vi "set_size.vi"(8 "error in (no error)":errorcluster, 10 "new size":refnum<class "SpaceVector.lvclass">, 11 "Box in":refnum<class "Box.lvclass">) -> (0 "error out":errorcluster, 3 "Box out":refnum<class "Box.lvclass">)   [LabVIEW 2010, in "Box.lvclass"]
uses:
  Box.lvclass
  SpaceVector/SpaceVector/SpaceVector.lvclass
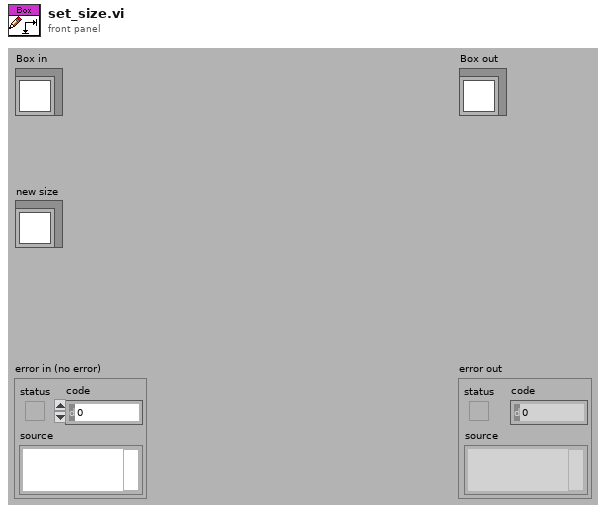
[diagram p1: front panel]
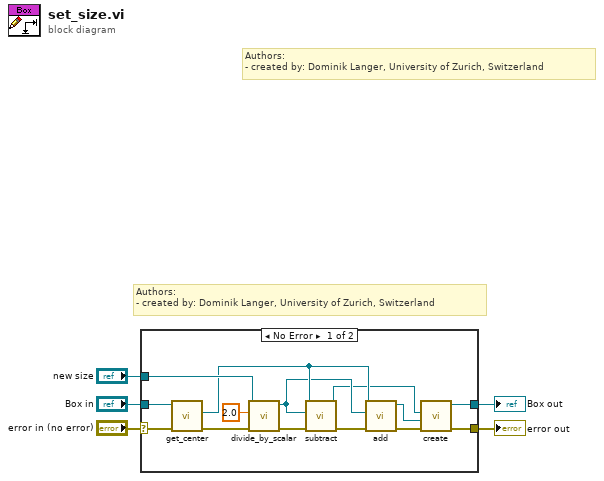
[diagram p0: block diagram]
diagram:
  # "Authors: \n- created by: Dominik Langer, University of Zurich, Switzerland"
  # "Authors: \n- created by: Dominik Langer, University of Zurich, Switzerland"
  n1 = case shown="No Error" "error in (no error)" {
    selector: "error in (no error)" -> [w18 w21]
    tunnel: [w9 w21] -> w4
    tunnel: [w6 w20] -> w2
    tunnel: "Box in" -> [w19 w20]
    tunnel: "new size" -> [w17 _]
    frame No Error {
      n2 = call "get_center.vi"("error in (no error)"=w18, "Box in"=w19) -> ("error out"=w16:errorcluster, "center"=w14:refnum<class "SpaceVector.lvclass">)  [unwired: 7 in, 1 out]
      n3 = call "divide_by_scalar.vi"("error in (no error)"=w16, "divisor"=2.0, "SpaceVector in"=w17) -> ("error out"=w13:errorcluster, "SpaceVector out"=w11:refnum<class "SpaceVector.lvclass">)  [unwired: 7 in]
      n4 = call "subtract.vi"("error in (no error)"=w13, "subtrahend"=w11, "SpaceVector in"=w14) -> ("error out"=w12:errorcluster, "SpaceVector out"=w7:refnum<class "SpaceVector.lvclass">)  [unwired: 7 in]
      n5 = call "add.vi"("error in (no error)"=w12, "vector to be added"=w11, "SpaceVector in"=w14) -> ("error out"=w10:errorcluster, "SpaceVector out"=w8:refnum<class "SpaceVector.lvclass">)  [unwired: 7 in]
      n6 = call "create.vi"("error in (no error)"=w10, "maximum"=w8, "minimum"=w7) -> ("error out"=w9:errorcluster, "Box out"=w6:refnum<class "Box.lvclass">)  [unwired: 7 in]
    }
    frame Error {
    }
  }
  "error out" <- w4
  "Box out" <- w2
